vi "Global_SEN Write_Data.vi"() -> ()   [LabVIEW 2017, in "System_Status.lvlib"]
uses:
  System_Status.lvlib
  TypeDef/CLUSTER_PDP_Status.ctl
  TypeDef/CLUSTER_PDP_Faults.ctl
  TypeDef/CLUSTER_PCM_Status.ctl
  _SHARE ALL/TypeDef Share All/CLUSTER_RoboRio_Status.ctl
  _SHARE ALL/TypeDef Share All/CLUSTER_RoboRio_Faults.ctl
  _SHARE ALL/TypeDef Share All/CLUSTER_RoboRio_Rails.ctl
  _SHARE ALL/TypeDef Share All/CLUSTER_RoboRio_SingleRail.ctl
panel:
  in  "SystemStatus_SEN_RoboRio":T1
  in  "SystemStatus_SEN_PCM":T5
  in  "SystemStatus_SEN_PDP":T6
  # "The Names of the Data items in the Global Variable MUST describe who the Single Writer is\nNaming Convention of all Data Items is:   Lib Name_Loop Name (SM or SEN or ACT)_Data Name\nExample   Drive_ACT_X axis;  GameController_SEN_JoystickLeft;  Hopper_SM_AgitatorSpeed"
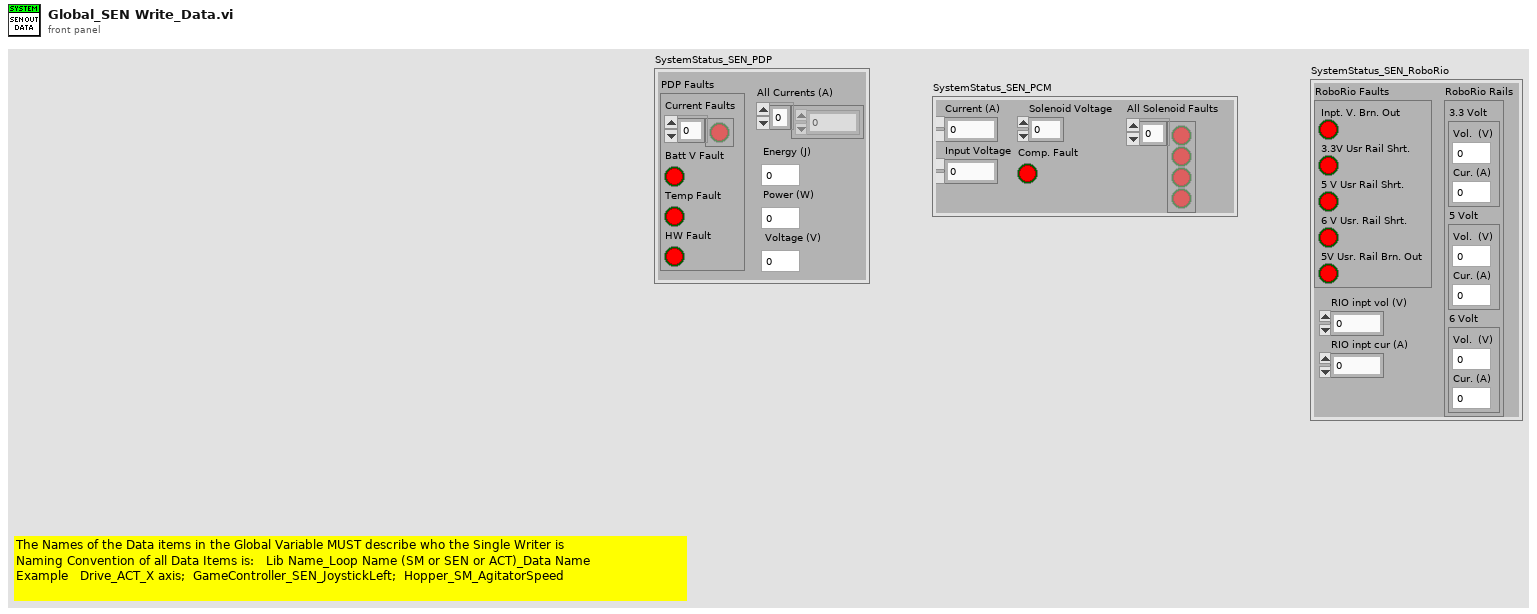
[diagram p1: front panel]
types:
  T1 = typedef "CLUSTER_RoboRio_Status.ctl" = cluster{"RoboRio Faults":T2, "RIO inpt vol (V)":dbl, "RIO inpt cur (A)":dbl, "RoboRio Rails":T3}
  T2 = typedef "CLUSTER_RoboRio_Faults.ctl" = cluster{"Inpt. V. Brn. Out":bool, "3.3V Usr Rail Shrt.":bool, "5 V Usr Rail Shrt.":bool, "6 V Usr. Rail Shrt.":bool, "5V Usr. Rail Brn. Out":bool}
  T3 = typedef "CLUSTER_RoboRio_Rails.ctl" = cluster{"3.3 Volt":T4, "5 Volt":T4, "6 Volt":T4}
  T4 = typedef "CLUSTER_RoboRio_SingleRail.ctl" = cluster{"Vol.  (V)":dbl, "Cur. (A)":dbl}
  T5 = typedef "CLUSTER_PCM_Status.ctl" = cluster{"Current (A)":dbl, "All Solenoid Faults":bool[], "Input Voltage":dbl, "Solenoid Voltage":dbl, "Comp. Fault":bool}
  T6 = typedef "CLUSTER_PDP_Status.ctl" = cluster{"PDP Faults":T7, "All Currents (A)":dbl[], "Energy (J)":dbl, "Power (W)":dbl, "Voltage (V)":dbl}
  T7 = typedef "CLUSTER_PDP_Faults.ctl" = cluster{"Current Faults":bool[], "Batt V Fault":bool, "Temp Fault":bool, "HW Fault":bool}
diagram:
